vi "Translate Weight Calibration 2.vi"() -> ()   [LabVIEW 2011]
uses:
  Shared Components/Config Manager Class/Type Definitions/Part Type.ctl
  Shared Components/Vec3d Class/Vec3d Class.lvclass
  Shared Components/Config Manager Class/Config Manager Class.lvclass
panel:
  out "brass piece rotation":dbl
  out "HDI XYZ":T1
  in  "Config Files Directory":path
  out "Weight XYZ":T2
  in  "weight start number":i32=1
  in  "PCA Config File":path
  out "Orient3d String":string
  out "Vec3d String":string
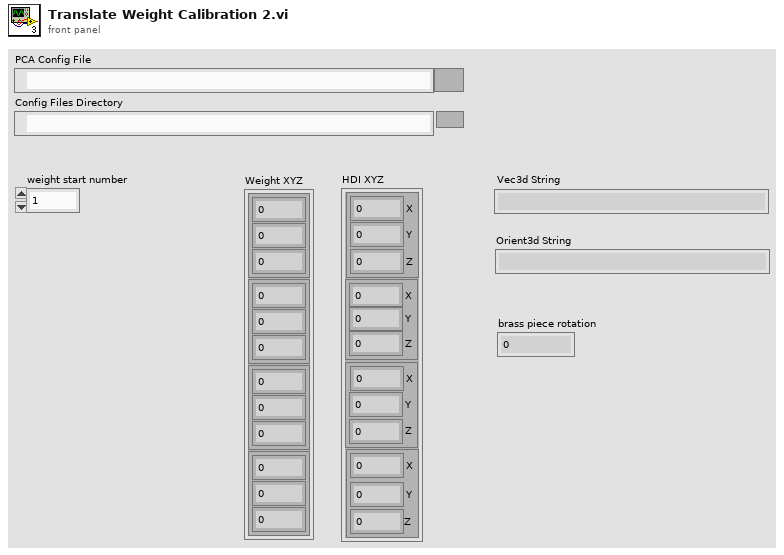
[diagram p1: front panel]
types:
  T1 = cluster{cluster{"X":dbl, "Y":dbl, "Z":dbl}, cluster{"X":dbl, "Y":dbl, "Z":dbl}, cluster{"X":dbl, "Y":dbl, "Z":dbl}, cluster{"X":dbl, "Y":dbl, "Z":dbl}}
  T2 = cluster{cluster{dbl, dbl, dbl}, cluster{dbl, dbl, dbl}, cluster{dbl, dbl, dbl}, cluster{dbl, dbl, dbl}}
  T3 = typedef "Part Type.ctl" = enum16{"BBM", "HDI", "BARE HDI", "GLUERESERVOIR", "STAMP_1", "STAMP_2", "STAMP_3", "STAMP_4", "STAMP_5", "WEIGHT_1", "WEIGHT_2", "WEIGHT_3", "WEIGHT_4", "WEIGHT_5", "WEIGHT_6", "WEIGHT_7", "WEIGHT_8", "PICKER_TOOL", "GRABER_TOOL"}
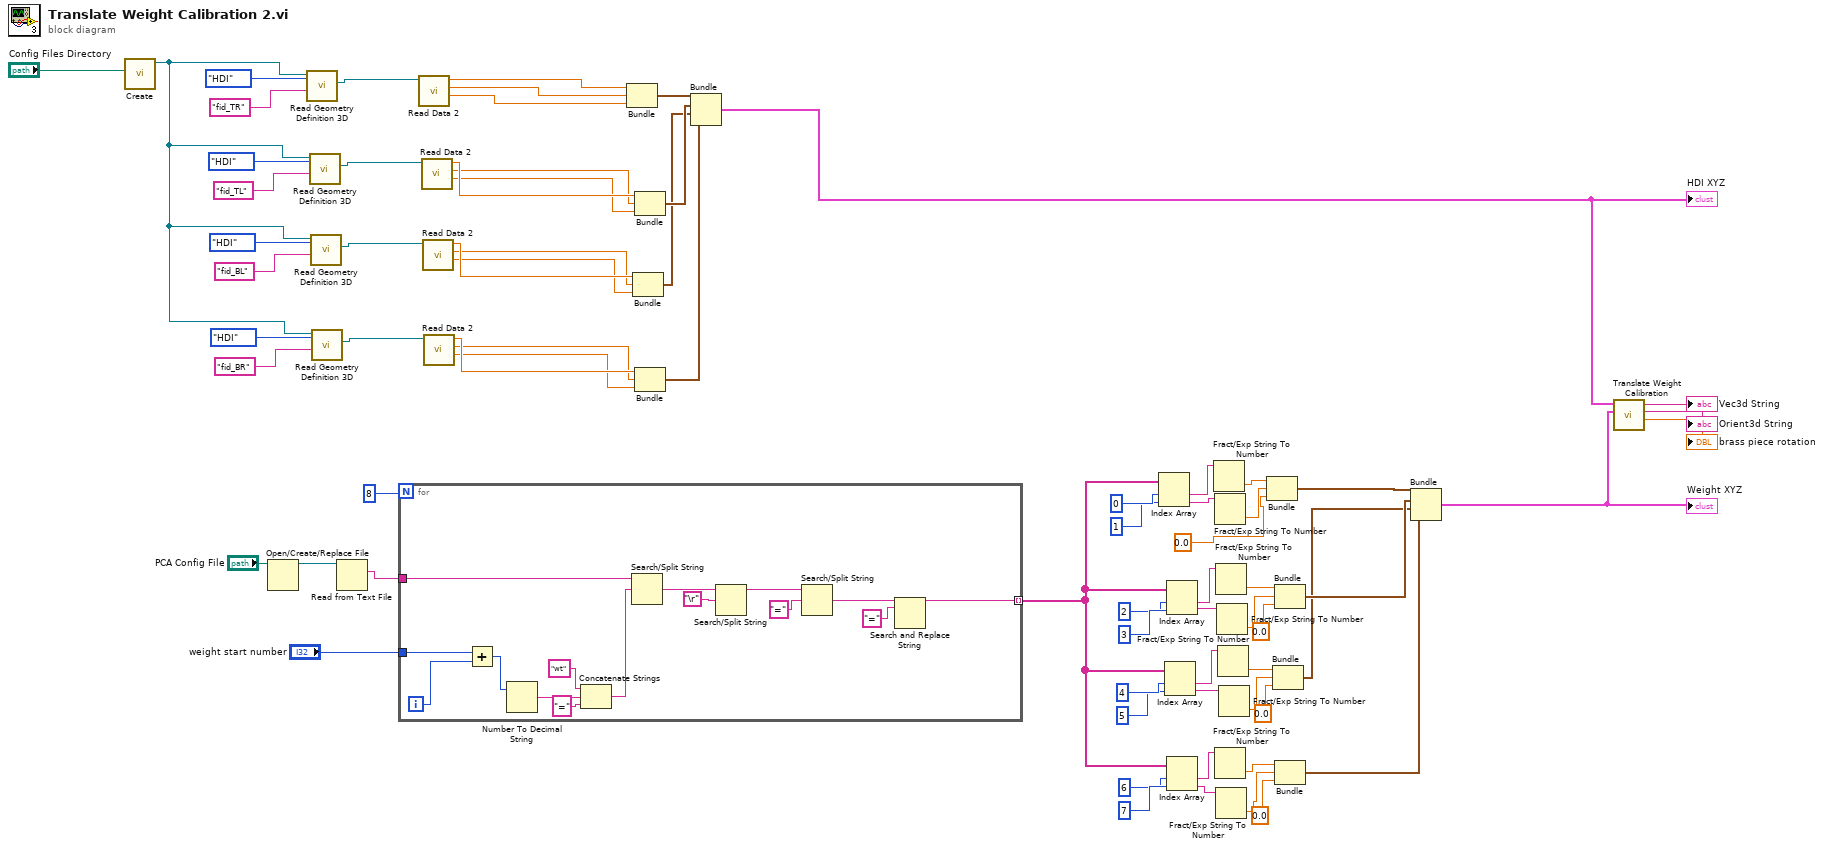
[diagram p0: block diagram]
diagram:
  n1 = call "Create.vi"("Config Files Directory"="Config Files Directory") -> ("Config Manager out"=w16:refnum<class "Config Manager Class.lvclass">)  [unwired: 9 in, 1 out]
  n2 = Open/Create/Replace File(file path (use dialog)="PCA Config File") -> (refnum out=w69:refnum<file>)  [unwired: 5 in, 2 out]
  n3 = call "Read Geometry Definition 3D.vi"("Feature"="fid_TR", "Part Type"=Part_Type."HDI", "Config Manager in"=w16) -> ("Feature Coordinates"=w29:refnum<class "Vec3d Class.lvclass">)  [unwired: 6 in, 2 out]
  n4 = call "Read Geometry Definition 3D.vi"("Feature"="fid_TL", "Part Type"=Part_Type."HDI", "Config Manager in"=w16) -> ("Feature Coordinates"=w25:refnum<class "Vec3d Class.lvclass">)  [unwired: 6 in, 2 out]
  n5 = call "Read Geometry Definition 3D.vi"("Feature"="fid_BL", "Part Type"=Part_Type."HDI", "Config Manager in"=w16) -> ("Feature Coordinates"=w20:refnum<class "Vec3d Class.lvclass">)  [unwired: 6 in, 2 out]
  n6 = call "Read Geometry Definition 3D.vi"("Feature"="fid_BR", "Part Type"=Part_Type."HDI", "Config Manager in"=w16) -> ("Feature Coordinates"=w19:refnum<class "Vec3d Class.lvclass">)  [unwired: 6 in, 2 out]
  n7 = Read from Text File(file (use dialog)=w69) -> (text=w68:string)  [unwired: 3 in, 3 out]
  n8 = for {
    N: 8 -> [_]
    tunnel: w68 -> [w78]
    tunnel: "weight start number" -> [w77]
    tunnel: [w74] -> w58 mode=indexing
    i -> [w76]
    n9 = Add(x=w77, y=w76) -> (x+y=w75:i32)
    n10 = Number To Decimal String(number=w75) -> (decimal integer string=w86:string)  [unwired: 1 in]
    n11 = Concatenate Strings("wt" ("string"), w86, "=" ("string")) -> (w88:string)
    n12 = Search/Split String(string=w78, search string/char (-)=w88) -> (match + rest of string=w79:string)  [unwired: 1 in, 2 out]
    n13 = Search/Split String(string=w79, search string/char (-)="\r") -> (substring before match=w82:string)  [unwired: 1 in, 2 out]
    n14 = Search/Split String(string=w82, search string/char (-)="=") -> (match + rest of string=w83:string)  [unwired: 1 in, 2 out]
    n15 = Search and Replace String(input string=w83, search string="=") -> (result string=w74:string)  [unwired: 6 in, 3 out]
  }
  n16 = call-dynamic "Read Data 2.vi"("Vec3d in"=w29) -> ("Z"=w12:dbl, "Y"=w27:dbl, "X"=w28:dbl)  [unwired: 7 in, 1 out]
  n17 = call-dynamic "Read Data 2.vi"("Vec3d in"=w25) -> ("Z"=w13:dbl, "Y"=w14:dbl, "X"=w15:dbl)  [unwired: 7 in, 1 out]
  n18 = call-dynamic "Read Data 2.vi"("Vec3d in"=w20) -> ("Z"=w9:dbl, "Y"=w10:dbl, "X"=w11:dbl)  [unwired: 7 in, 1 out]
  n19 = call-dynamic "Read Data 2.vi"("Vec3d in"=w19) -> ("Z"=w6:dbl, "Y"=w7:dbl, "X"=w8:dbl)  [unwired: 7 in, 1 out]
  n20 = Bundle("X"=w28, "Y"=w27, "Z"=w12) -> (w26:cluster{"X":dbl, "Y":dbl, "Z":dbl})  [unwired: 1 in]
  n21 = Bundle("X"=w11, "Y"=w10, "Z"=w9) -> (w4:cluster{"X":dbl, "Y":dbl, "Z":dbl})  [unwired: 1 in]
  n22 = Bundle("X"=w15, "Y"=w14, "Z"=w13) -> (w5:cluster{"X":dbl, "Y":dbl, "Z":dbl})  [unwired: 1 in]
  n23 = Bundle("X"=w8, "Y"=w7, "Z"=w6) -> (w3:cluster{"X":dbl, "Y":dbl, "Z":dbl})  [unwired: 1 in]
  n24 = Bundle(w26, w5, w4, w3) -> (w2:T1)  [unwired: 1 in]
  "HDI XYZ" <- w2
  n25 = Index Array(array=w58, index #1=0 ("index"), index #2=1 ("index")) -> (element #1=w52:string, element #2=w50:string)
  n26 = Index Array(array=w58, index #1=4 ("index"), index #2=5 ("index")) -> (element #1=w41:string, element #2=w42:string)
  n27 = Index Array(array=w58, index #1=2 ("index"), index #2=3 ("index")) -> (element #1=w44:string, element #2=w43:string)
  n28 = Index Array(array=w58, index #1=6 ("index"), index #2=7 ("index")) -> (element #1=w36:string, element #2=w37:string)
  n29 = Fract/Exp String To Number(string=w52) -> (number=w51:dbl)  [unwired: 3 in, 1 out]
  n30 = Fract/Exp String To Number(string=w50) -> (number=w49:dbl)  [unwired: 3 in, 1 out]
  n31 = Fract/Exp String To Number(string=w36) -> (number=w35:dbl)  [unwired: 3 in, 1 out]
  n32 = Fract/Exp String To Number(string=w44) -> (number=w46:dbl)  [unwired: 3 in, 1 out]
  n33 = Fract/Exp String To Number(string=w37) -> (number=w33:dbl)  [unwired: 3 in, 1 out]
  n34 = Fract/Exp String To Number(string=w43) -> (number=w47:dbl)  [unwired: 3 in, 1 out]
  n35 = Fract/Exp String To Number(string=w41) -> (number=w40:dbl)  [unwired: 3 in, 1 out]
  n36 = Fract/Exp String To Number(string=w42) -> (number=w39:dbl)  [unwired: 3 in, 1 out]
  n37 = Bundle(w51, w49, 0.0) -> (w53:cluster{dbl, dbl, dbl})  [unwired: 1 in]
  n38 = Bundle(w40, w39, 0.0) -> (w56:cluster{dbl, dbl, dbl})  [unwired: 1 in]
  n39 = Bundle(w46, w47, 0.0) -> (w57:cluster{dbl, dbl, dbl})  [unwired: 1 in]
  n40 = Bundle(w35, w33, 0.0) -> (w55:cluster{dbl, dbl, dbl})  [unwired: 1 in]
  n41 = Bundle(w53, w57, w56, w55) -> (w54:T2)  [unwired: 1 in]
  "Weight XYZ" <- w54
  n42 = call "Translate Weight Calibration.vi"("Known Weight Tool Coordinates"=w54, "Known HDI Fiducials Coordinates"=w2) -> ("brass piece rotation"=→"brass piece rotation":dbl, "Orient3d String"=→"Orient3d String":string, "Vec3d String"=→"Vec3d String":string)  [unwired: 7 in]
